vi "16 K MULTIRAM chip.vi"(1 "Clock":bool, 2 "Address'":bool[][](array[boolean]), 3 "Data In":bool[][](array[boolean]), 4 "Hold":bool) -> (0 "Registers Out":bool[][](array[boolean]))   [LabVIEW 2012]
panel:
  in  "Destination Address'":bool[][](array[boolean])
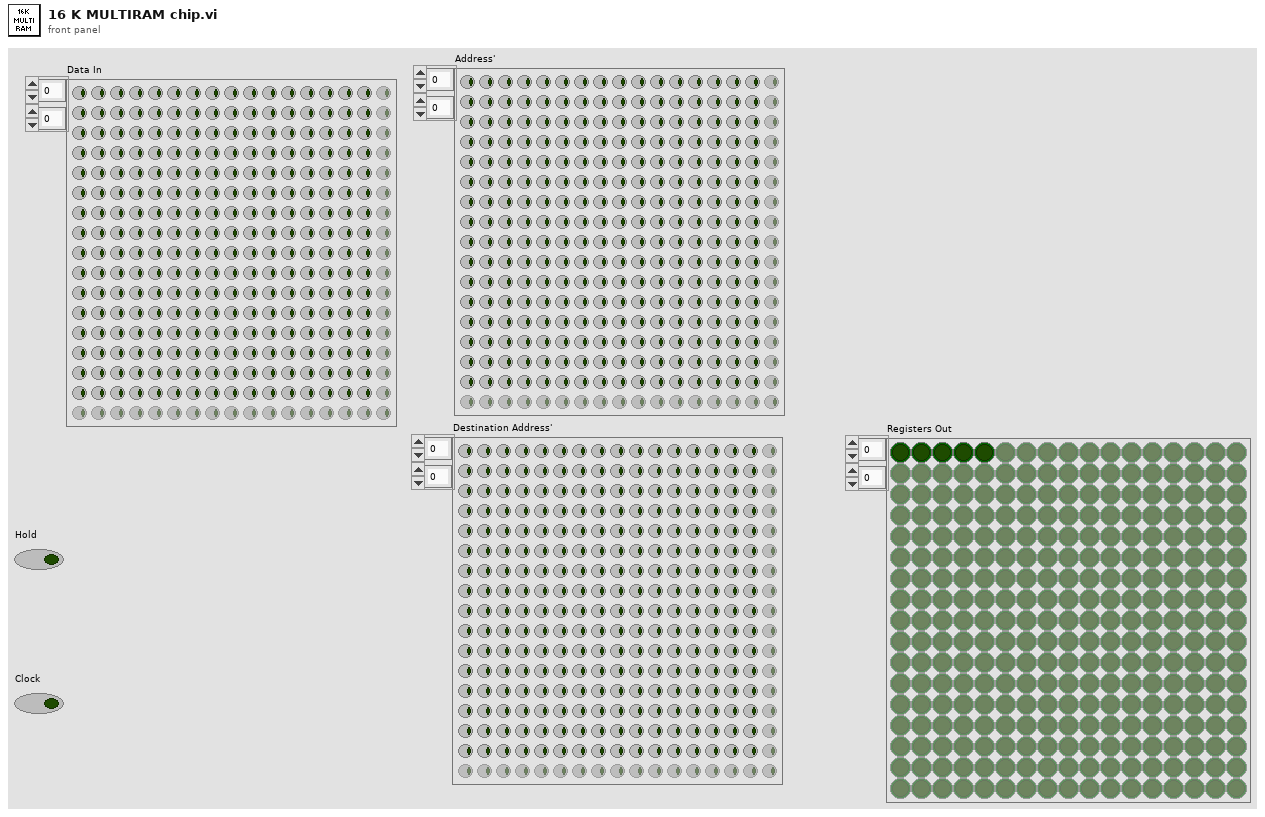
[diagram p1: front panel]
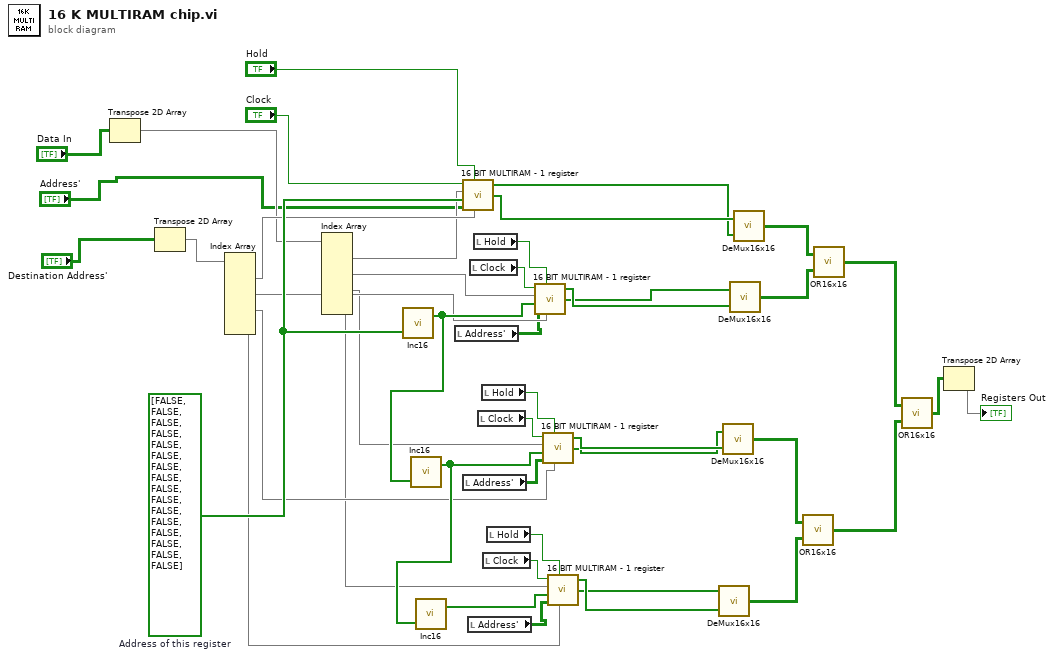
[diagram p0: block diagram]
diagram:
  w44 = bool[] [FALSE, FALSE, FALSE, FALSE, FALSE, FALSE, FALSE, FALSE, FALSE, FALSE, FALSE, FALSE, FALSE, FALSE, FALSE, FALSE]  # Address of this register
  n1 = Transpose 2D Array(2D array="Data In") -> (transposed array=w9:bool[][])
  n2 = Transpose 2D Array(2D array="Destination Address'") -> (transposed array=w8:bool[][])
  n3 = Index Array(array=w8) -> (element #1=w32:bool[], element #2=w31:bool[], element #3=w30:bool[], element #4=w29:bool[])  [unwired: 8 in]
  n4 = Index Array(array=w9) -> (element #1=w14:bool[], element #2=w13:bool[], element #3=w12:bool[], element #4=w11:bool[])  [unwired: 8 in]
  n5 = call "Inc16.vi"("A"=w44) -> ("S"=w37:bool[])  [unwired: 1 in, 1 out]
  n6 = call "Inc16.vi"("A"=w37) -> ("S"=w33:bool[])  [unwired: 1 in, 1 out]
  n7 = call "Inc16.vi"("A"=w33) -> ("S"=w34:bool[])  [unwired: 1 in, 1 out]
  n8 = local read "Address'"() -> (w6:bool[][])
  n9 = call "16 BIT MULTIRAM - 1 register.vi"("Clock"="Clock", "Hold"="Hold", "Data In"=w14, "Address of this register"=w44, "Destination Address In"=w32, "Address'"="Address'") -> ("z"=w27:bool[], "Destination Address Out"=w28:bool[])  [unwired: 1 out]
  n10 = local read "Address'"() -> (w5:bool[][])
  n11 = local read "Address'"() -> (w4:bool[][])
  n12 = local read "Clock"() -> (w40:bool)
  n13 = local read "Hold"() -> (w41:bool)
  n14 = local read "Clock"() -> (w39:bool)
  n15 = local read "Hold"() -> (w38:bool)
  n16 = local read "Clock"() -> (w35:bool)
  n17 = local read "Hold"() -> (w36:bool)
  n18 = call "16 BIT MULTIRAM - 1 register.vi"("Clock"=w40, "Hold"=w41, "Data In"=w13, "Address of this register"=w37, "Destination Address In"=w31, "Address'"=w6) -> ("z"=w26:bool[], "Destination Address Out"=w23:bool[])  [unwired: 1 out]
  n19 = call "16 BIT MULTIRAM - 1 register.vi"("Clock"=w39, "Hold"=w38, "Data In"=w12, "Address of this register"=w33, "Destination Address In"=w30, "Address'"=w5) -> ("z"=w25:bool[], "Destination Address Out"=w22:bool[])  [unwired: 1 out]
  n20 = call "16 BIT MULTIRAM - 1 register.vi"("Clock"=w35, "Hold"=w36, "Data In"=w11, "Address of this register"=w34, "Destination Address In"=w29, "Address'"=w4) -> ("z"=w24:bool[], "Destination Address Out"=w21:bool[])  [unwired: 1 out]
  n21 = call "DeMux16x16.vi"("Data"=w24, "Select"=w21) -> ("A"=w17:bool[][])
  n22 = call "DeMux16x16.vi"("Data"=w25, "Select"=w22) -> ("A"=w18:bool[][])
  n23 = call "DeMux16x16.vi"("Data"=w26, "Select"=w23) -> ("A"=w19:bool[][])
  n24 = call "DeMux16x16.vi"("Data"=w27, "Select"=w28) -> ("A"=w20:bool[][])
  n25 = call "OR16x16.vi"("B"=w17, "A"=w18) -> ("z"=w16:bool[][])
  n26 = call "OR16x16.vi"("B"=w19, "A"=w20) -> ("z"=w15:bool[][])
  n27 = call "OR16x16.vi"("B"=w16, "A"=w15) -> ("z"=w2:bool[][])
  n28 = Transpose 2D Array(2D array=w2) -> (transposed array=→"Registers Out":bool[][])
